vi "Get Value.vi"(8 "error in (no error)":errorcluster, 11 "Element A in":refnum<class "Element B.lvclass">) -> (0 "error out":errorcluster, 2 "Value":string, 3 "Element A out":refnum<class "Element B.lvclass">)   [LabVIEW 2020, in "Array Example.lvlib" / "Element B.lvclass"]
uses:
  Element B.lvclass
  Element B.lvclass/Element B.ctl
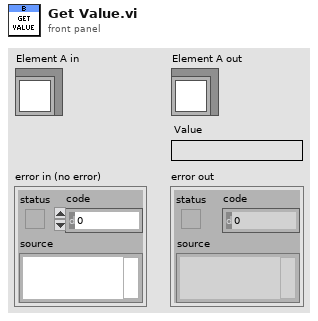
[diagram p1: front panel]
types:
  T1 = typedef "Element B.lvclass/Ref.ctl" = cluster{"Value":dbl}
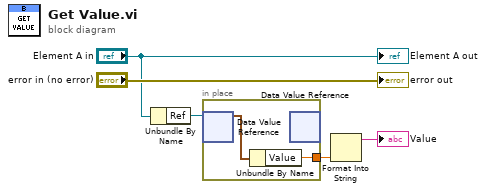
[diagram p0: block diagram]
diagram:
  n1 = Unbundle By Name("Element A in") -> ("Ref"=w4:refnum<data-value>)
  n2 = in-place {
    in-place-border: [w6] -> w2
    n3 = in-place-dvr #1(w4) -> (w7:T1)  [unwired: 1 out]
    n4 = Unbundle By Name(w7) -> ("Value"=w6:dbl)
    n5 = in-place-dvr #1() -> ()  [unwired: 1 in, 2 out]
  }
  n6 = Format Into String(w2) -> (resulting string=→"Value":string)  [unwired: 3 in, 1 out]
  "error out" <- "error in (no error)"
  "Element A out" <- "Element A in"
